vi "Instrument Command Response.vi"(8 "error in (no error)":errorcluster, 10 "Command Parameters":T2, 11 "connection info":T4) -> (0 "error out":errorcluster, 1 "Timed Out?":bool, 2 "Response":T1, 3 "connection info":T4)   [LabVIEW 2019, in "Instrument CD Host API.lvlib"]
uses:
  Instrument CD Host API.lvlib
  <vilib>/NI/STM/TCP/TCP Connection Info.ctl
  <vilib>/NI/STM/SubVIs/MetaDataElement.ctl
  Engine/Types/Buffered RT Instrument Command.ctl
  Shared/Types/Response Wait Type.ctl
  Engine/Types/Buffered RT Instrument Request.ctl
  Engine/Instrument Addon Engine.lvlib
  <vilib>/NI/NIVS Addon Network Comm/Shared/NI VeriStand Addon Network Comm Shared.lvlib
  Shared/Instrument Addon Shared.lvlib
  <vilib>/NI/STM/NI STM.lvlib
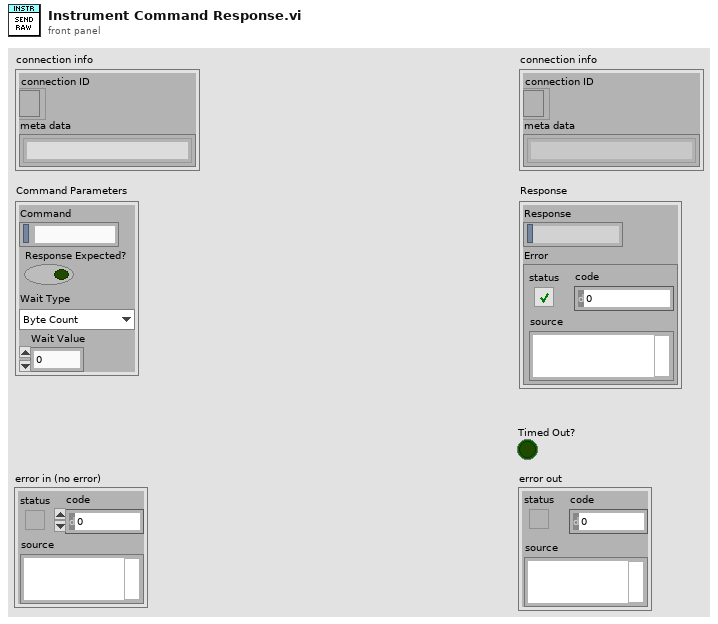
[diagram p1: front panel]
types:
  T1 = typedef "Instrument Addon Engine.lvlib/Buffered RT Instrument Request.ctl" = cluster{"Response":string, "Error":errorcluster}
  T2 = typedef "Instrument Addon Engine.lvlib/Buffered RT Instrument Command.ctl" = cluster{"Command":string, "Response Expected?":bool, "Wait Type":T3, "Wait Value":dbl}
  T3 = typedef "Instrument Addon Shared.lvlib/Response Wait Type.ctl" = enum16{"Byte Count", "Wait sec"}
  T4 = typedef "NI STM.lvlib/TCP Connection Info.ctl" = cluster{"connection ID":refnum<k5>, "meta data":T5[]}
  T5 = typedef "NI STM.lvlib/MetaDataElement.ctl" = string
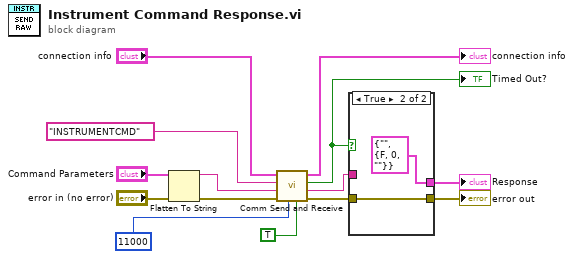
[diagram p0: block diagram]
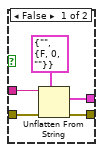
[diagram p2: hidden frame]
diagram:
  n1 = Flatten To String(anything="Command Parameters", error in (no error)="error in (no error)") -> (data string=w3:string, error out=w9:errorcluster)  [unwired: 2 in, 1 out]
  n2 = call <vilib>:"Comm Send and Receive.vi"("Resp Required?"=TRUE, "Timeout (ms)"=u32 11000, "error in (no error)"=w9, "Data"=w3, "Name"="INSTRUMENTCMD", "connection info"="connection info") -> ("error out"=w7:errorcluster, "Data"=w8:string, "Timed Out?"=w2:bool, "connection info"=→"connection info":T4)  [unwired: 2 in]
  "Timed Out?" <- w2
  n3 = case shown="True" w2 {
    tunnel: w8 -> [w19 _]
    tunnel: w7 -> [w18 w21]
    tunnel: [w17 w21] -> w6
    tunnel: [w15 T1 {"Response"="", "Error"={"status"=FALSE, "code"=0, "source"=""}} ("Cluster")] -> w5
    frame False {
      n4 = Unflatten From String(type=T1 {"Response"="", "Error"={"status"=FALSE, "code"=0, "source"=""}} ("Cluster"), binary string=w19, error in (no error)=w18) -> (value=w15:T1, error out=w17:errorcluster)  [unwired: 2 in, 1 out]
    }
    frame True {
    }
  }
  "error out" <- w6
  "Response" <- w5
